vi "WILT Panel Update Dryer Details.vi"(0 "Dryer Details In":T1) -> (4 "Dryer Details Out":T1, 6 "New Filenames":bool, 8 "Updated":bool)   [LabVIEW 2016]
uses:
  Type Definitions/WILT Dryer Details.ctl
panel:
  in  "Tab Control":enum32{"Update Panel", "Debug"}(tab)
  in  "Stop Dryer":i32(ring) items=["NO", "YES"]
  in  "24 Hour Water Injection":i32(ring) items=["NO", "YES"]
  in  "Run w/o Newfi":i32(ring) items=["NO", "YES"]
  out "Station":string
  in  "Lab ID":string
  in  "Notes":string
  in  "TR Number":string
  in  "stop":bool
  in  "Cycle Count Day":string
  in  "Cycle Count Night":string
  in  "Time On Day":string
  in  "Time On Night":string
  in  "Cancel":bool
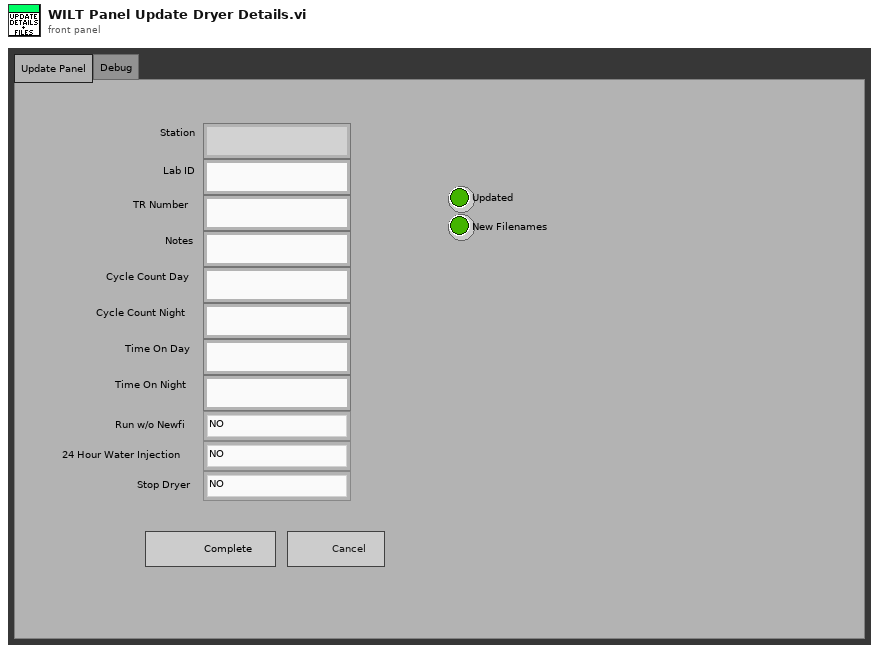
[diagram p1: front panel]
types:
  T1 = typedef "WILT Dryer Details.ctl" = cluster{"Station":string, "Lab ID":string, "TR Number":string}
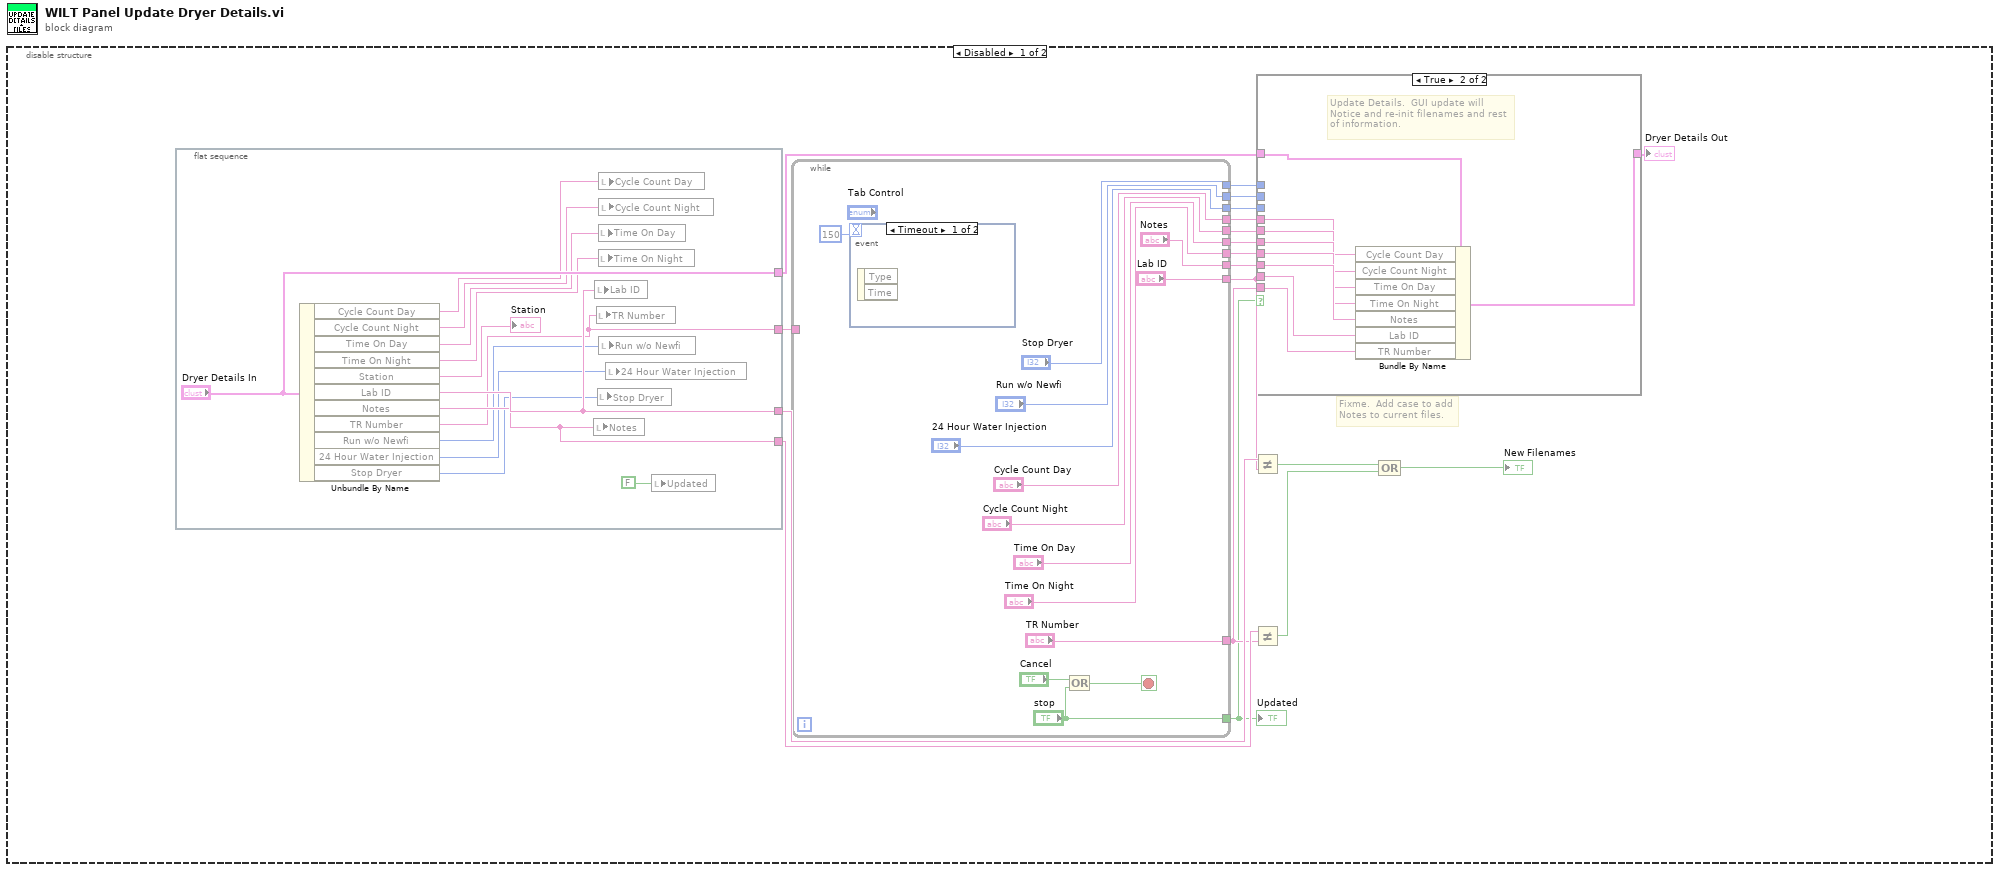
[diagram p0: block diagram]
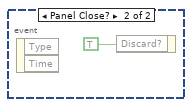
[diagram p3: hidden frame]
diagram:
  n1 = disable-structure shown="Disabled" {
    frame Disabled {
      # "Fixme.  Add case to add\nNotes to current files."
      n2 = flat-sequence {
        tunnel: [w39] -> w19
        tunnel: [w41] -> w16
        tunnel: [w40] -> w15
        tunnel: ["Dryer Details In"] -> w10
        frame #0 {
          n3 = Unbundle By Name("Dryer Details In") -> ("Cycle Count Day"=w34:string, "Cycle Count Night"=w35:string, "Time On Day"=w36:string, "Time On Night"=w37:string, "Station"=→"Station":string, "Lab ID"=w41:string, "Notes"=w40:string, "TR Number"=w39:string, "Run w/o Newfi"=w32:i32, "24 Hour Water Injection"=w33:i32, "Stop Dryer"=w31:i32)
          n4 = local write "Notes"(w40) -> ()
          n5 = local write "Lab ID"(w41) -> ()
          n6 = local write "TR Number"(w39) -> ()
          n7 = local write "Stop Dryer"(w31) -> ()
          n8 = local write "Time On Day"(w36) -> ()
          n9 = local write "Time On Night"(w37) -> ()
          n10 = local write "Cycle Count Day"(w34) -> ()
          n11 = local write "Cycle Count Night"(w35) -> ()
          n12 = local write "Run w/o Newfi"(w32) -> ()
          n13 = local write "24 Hour Water Injection"(w33) -> ()
          n14 = local write "Updated"(FALSE ("Updated")) -> ()
        }
      }
      n15 = while {
        tunnel: w19 -> [_]
        tunnel: ["Lab ID"] -> w12
        tunnel: ["TR Number"] -> w13
        tunnel: ["Notes"] -> w11
        tunnel: ["Time On Night"] -> w8
        tunnel: ["Time On Day"] -> w7
        tunnel: ["Cycle Count Night"] -> w6
        tunnel: ["Cycle Count Day"] -> w5
        tunnel: ["stop"] -> w4
        tunnel: ["Run w/o Newfi"] -> w3
        tunnel: ["24 Hour Water Injection"] -> w2
        tunnel: ["Stop Dryer"] -> w1
        stop <- w48 stop-if-true
        n16 = event shown="[0] Timeout" {
          selector: _ -> [_ _]
          dyn-events: _ -> [_ _]
          timeout: 150 ("milliseconds to wait") -> [_ _]
          event Timeout {
            n17 = event-data() -> ()  [unwired: 1 in, 2 out]
          }
          event Panel Close? {
            n18 = event-data() -> ()  [unwired: 1 in, 2 out]
            n19 = event-data("Discard?"=TRUE) -> ()  [unwired: 1 in, 1 out]
          }
        }
        n20 = Or(x="Cancel", y="stop") -> (x .or. y?=w48:bool)
      }
      "Updated" <- w4
      n21 = Not Equal?(x=w16, y=w12) -> (x != y?=w18:bool)
      n22 = Not Equal?(x=w15, y=w13) -> (x != y?=w17:bool)
      n23 = case shown="True" w4 {
        tunnel: w13 -> [_ w26]
        tunnel: w12 -> [_ w25]
        tunnel: w11 -> [_ w28]
        tunnel: w10 -> [w20 w29]
        tunnel: [w20 w27] -> w9
        tunnel: w8 -> [_ w24]
        tunnel: w7 -> [_ w23]
        tunnel: w6 -> [_ w22]
        tunnel: w5 -> [_ w21]
        tunnel: w3 -> [_ _]
        tunnel: w2 -> [_ _]
        tunnel: w1 -> [_ _]
        frame False {
        }
        frame True {
          # "Update Details.  GUI update will\nNotice and re-init filenames and rest\nof information."
          n24 = Bundle By Name(cluster=w29, "Cycle Count Day"=w21, "Cycle Count Night"=w22, "Time On Day"=w23, "Time On Night"=w24, "Notes"=w28, "Lab ID"=w25, "TR Number"=w26) -> (w27:T1)
        }
      }
      "Dryer Details Out" <- w9
      n25 = Compound Arithmetic op=OR(w18, w17) -> (→"New Filenames":bool)
    }
    frame Enabled {
    }
  }
